vi "Process Image.vi"(8 "error in (no error)":errorcluster, 9 "Processed Frames per Second":dbl, 10 "Image In":T1, 11 "CameraPreview in":refnum<class "CameraPreview.lvclass">) -> (0 "error out":errorcluster, 3 "CameraPreview out":refnum<class "CameraPreview.lvclass">)   [LabVIEW 2023, in "CameraPreview.lvlib" / "CameraPreview.lvclass"]
uses:
  CameraPreview.lvclass
  CameraPreview.lvclass/CameraPreview.ctl
  <vilib>/vision/NI_Vision_Development_Module.lvlib
  Camera_Controller/Camera_Controller.lvlib
  Interfaces/AbstractInstrumentClasses/Cameras_LV/CameraComm Messages/Frame Ready Msg/Frame Ready Msg.lvclass
  <vilib>/ActorFramework/Actor/Actor.lvclass
  C:/Program Files/National Instruments/LabVIEW 2023/vi.lib/ActorFramework/Actor/Actor.lvclass
  C:/Users/quantum/Documents/LVDAQ/UIs/Camera_Preview/CameraPreview/CameraPreview/CameraPreview.lvclass
  <vilib>/vision/Image Controls.llb/IMAQ Image.ctl
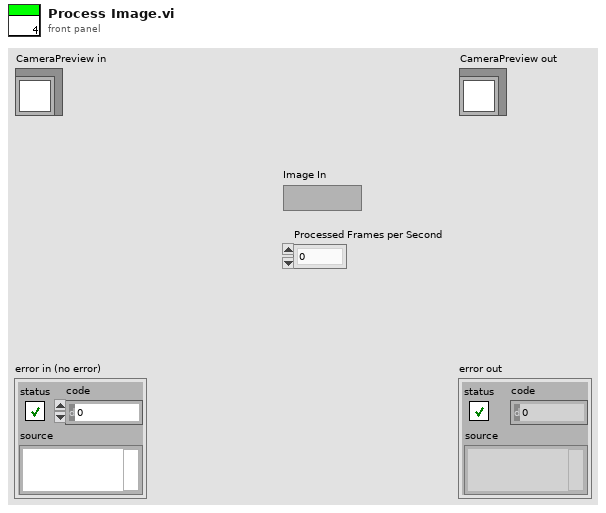
[diagram p1: front panel]
types:
  T1 = typedef "IMAQ Image.ctl" = refnum<image>
  T2 = enum32{"Linear", "Log", "Exp", "Square", "Square root", "Power X", "Power 1/X"}
  T3 = cluster{"Brightness":sgl, "Contrast":sgl, "Gamma":sgl}
  T4 = cluster{"Lower value":sgl, "Upper value":sgl, "Replace Value":sgl, "Keep/Replace Value (Replace)":bool}[]
  T5 = cluster{"Global Rectangle":i32[], "Contours":cluster{"Contour Type":u32, "ROI Type":u32, "Points":i32[]}[]}
  T6 = cluster{"Min":sgl, "Max":sgl, "Mean":sgl, "Std Dev":sgl, "Count":i32, "Size (um)":i32}
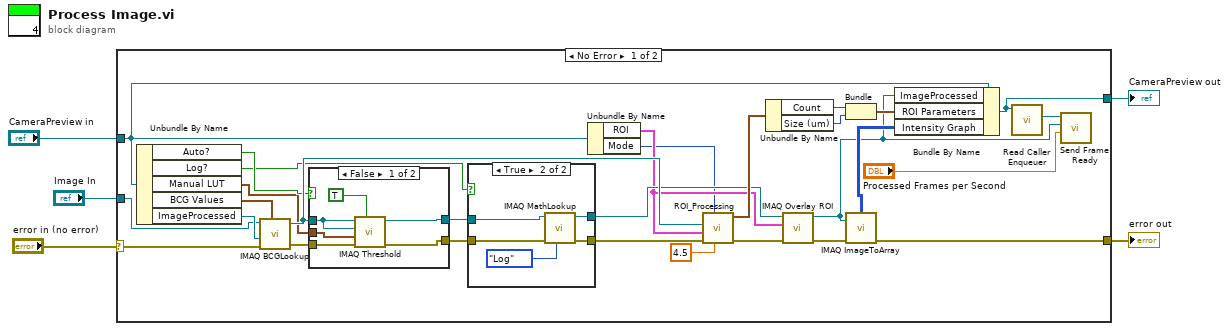
[diagram p0: block diagram]
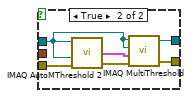
[diagram p3: hidden frame]
diagram:
  n1 = case shown="No Error" "error in (no error)" {
    selector: "error in (no error)" -> [w14 w55]
    tunnel: [w13 w55] -> w4
    tunnel: [w10 w54] -> w2
    tunnel: "CameraPreview in" -> [w12 w54]
    tunnel: "Image In" -> [w15 _]
    frame No Error {
      n2 = Unbundle By Name(w12) -> ("Auto?"=w26:bool, "Log?"=w23:bool, "Manual LUT"=w25:cluster{"Minimum":dbl, "Maximum":dbl}, "BCG Values"=w24:T3, "ImageProcessed"=w16:T1)
      n3 = call "IMAQ BCGLookup"("Image Src"=w15, "BCG Values"=w24, "Image Dst"=w16, "error in (no error)"=w14) -> ("Image Dst Out"=w33:T1, "error out"=w32:errorcluster)  [unwired: 3 in]
      n4 = case shown="False" w26 {
        tunnel: w33 -> [w43 w51]
        tunnel: [w45 w50] -> w30
        tunnel: w32 -> [w47 w53]
        tunnel: [w46 w48] -> w31
        tunnel: w25 -> [w44 _]
        frame False {
          n5 = call "IMAQ Threshold"("Keep/Replace Value (Replace)"=TRUE, "error in (no error)"=w47, "Range"=w44, "Image Dst"=w43, "Image Src"=w43) -> ("error out"=w46:errorcluster, "Image Dst Out"=w45:T1)  [unwired: 5 in]
        }
        frame True {
          n6 = call "IMAQ AutoMThreshold 2"("error in (no error)"=w53, "Image Mask"=w51, "Image"=w51) -> ("error out"=w49:errorcluster, "Threshold Data out"=w52:T4)  [unwired: 1 in, 1 out]
          n7 = call "IMAQ MultiThreshold"("error in (no error)"=w49, "Threshold Data"=w52, "Image Dst"=w51, "Image Src"=w51) -> ("error out"=w48:errorcluster, "Image Dst Out"=w50:T1)  [unwired: 1 in]
        }
      }
      n8 = case shown="True" w23 {
        tunnel: w30 -> [w35 w40]
        tunnel: w31 -> [w36 w39]
        tunnel: [w36 w38] -> w22
        tunnel: [w35 w37] -> w21
        frame False {
        }
        frame True {
          n9 = call "IMAQ MathLookup"("Operator"=T2."Log", "error in (no error)"=w39, "Image Src"=w40) -> ("error out"=w38:errorcluster, "Image Dst Out"=w37:T1)  [unwired: 7 in]
        }
      }
      n10 = Unbundle By Name(w12) -> ("ROI"=w18:T5, "Mode"=w17:enum16{"ROI", "Image"})
      n11 = call "ROI_Processing.vi"("Pixel Size(um)"=4.5, "Histogram Mode"=w17, "error in (no error)"=w22, "ROI"=w18, "Image Dst Out"=w33) -> ("error out"=w20:errorcluster, "ROI Pixel Statistics"=w27:T6)  [unwired: 4 in, 1 out]
      n12 = Unbundle By Name(w27) -> ("Count"=w28:i32, "Size (um)"=w29:i32)
      n13 = call "IMAQ Overlay ROI"("error in (no error)"=w20, "ROI Descriptor"=w18, "Image"=w21) -> ("error out"=w19:errorcluster, "Image Out"=w6:T1)  [unwired: 7 in]
      n14 = Bundle("Count"=w28, "Size (um)"=w29) -> (w8:cluster{"Count":i32, "Size (um)":i32})  [unwired: 1 in]
      n15 = call "IMAQ ImageToArray"("error in (no error)"=w19, "Image"=w6) -> ("error out"=w13:errorcluster, "Image Pixels (U8)"=w9:u8[][])  [unwired: 2 in, 3 out]
      n16 = Bundle By Name(cluster=w12, "ImageProcessed"=w6, "ROI Parameters"=w8, "Intensity Graph"=w9) -> (w10:refnum<class "CameraPreview.lvclass">)
      n17 = call <vilib>:"Read Caller Enqueuer.vi"("Actor"=w10) -> ("Caller Enqueuer"=w11:refnum<class "Message Enqueuer.lvclass">)  [unwired: 10 in]
      n18 = call "Send Frame Ready.vi"("Processed Frames per Second"="Processed Frames per Second", "Image In"=w6, "Message Enqueuer"=w11) -> ()  [unwired: 7 in, 2 out]
    }
    frame Error {
    }
  }
  "error out" <- w4
  "CameraPreview out" <- w2
